vi "TagMetadataToImage.vi"(8 "error in (no error)":errorcluster, 10 "Image In":T1, 11 "Stage_MadCityLab in":refnum<class "Stage_MadCityLab.lvclass">) -> (0 "error out":errorcluster, 2 "Image Out":T1, 3 "Stage_MadCityLab out":refnum<class "Stage_MadCityLab.lvclass">)   [LabVIEW 2020, in "Stage_MadCityLab.lvlib" / "Stage_MadCityLab.lvclass"]
uses:
  Stage_MadCityLab.lvclass
  <vilib>/ActorFramework/Actor/Actor.lvclass
  <vilib>/vision/Image Controls.llb/IMAQ Image.ctl
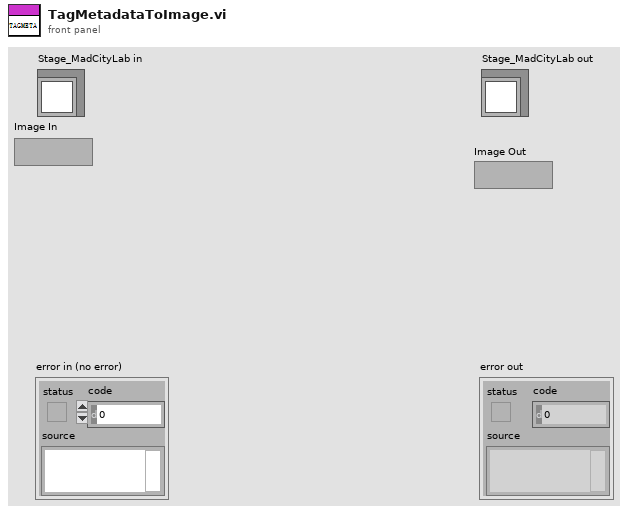
[diagram p1: front panel]
types:
  T1 = typedef "IMAQ Image.ctl" = refnum<image>
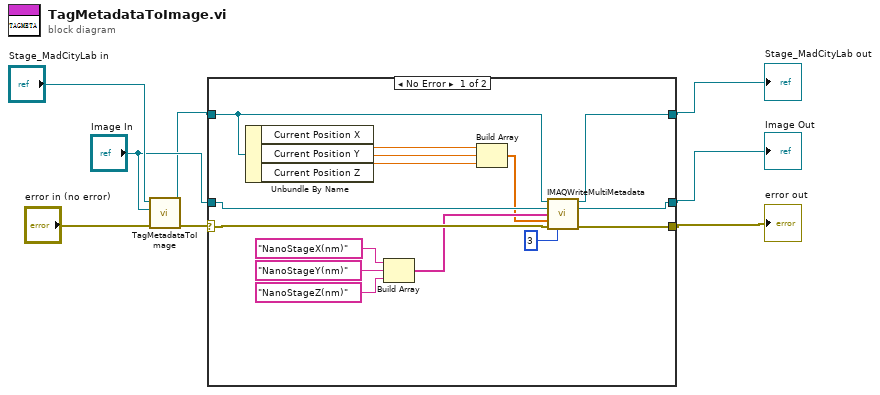
[diagram p0: block diagram]
diagram:
  n1 = call-parent "TagMetadataToImage.vi"("error in (no error)"="error in (no error)", "Image In"="Image In", "Device in"="Stage_MadCityLab in") -> ("error out"=w6:errorcluster, "Device out"=w4:refnum<class "Stage_MadCityLab.lvclass">)  [unwired: 6 in, 1 out]
  n2 = case shown="No Error" w6 {
    selector: w6 -> [w23 w26]
    tunnel: [w21 w26] -> w3
    tunnel: "Image In" -> [w22 w24]
    tunnel: [w20 w25] -> w1
    tunnel: w4 -> [w10 w25]
    tunnel: [w19 w24] -> w2
    frame No Error {
      n3 = Unbundle By Name(w10) -> ("Current Position X"=w13:dbl, "Current Position Y"=w12:dbl, "Current Position Z"=w11:dbl)
      n4 = Build Array("NanoStageX(nm)" ("Key"), "NanoStageY(nm)" ("Key"), "NanoStageZ(nm)" ("Key")) -> (w14:string[])
      n5 = Build Array(w13, w12, w11) -> (w9:dbl[])
      n6 = call-dynamic "IMAQWriteMultiMetadata.vi"("GRMActor in"=w10, "Image In"=w22, "Keys"=w14, "Values"=w9, "error in (no error)"=w23, "precision (6)"=i16 3) -> ("GRMActor out"=w20:refnum<class "Stage_MadCityLab.lvclass">, "Image Out"=w19:T1, "error out"=w21:errorcluster)  [unwired: 7 in]
    }
    frame Error {
    }
  }
  "error out" <- w3
  "Stage_MadCityLab out" <- w1
  "Image Out" <- w2
